vi "PCO_squeeze_puff_pupil_FLIR_trig_2024_JMR.vi"() -> ()   [LabVIEW 2020]
uses:
  C:/Users/jqr5792/AppData/Roaming/PCO Digital Camera Toolbox/pco.labview/pco.camera/Controls/binning.ctl
  <vilib>/vision/driver/IMAQdx.llb/IMAQdx Camera Control Mode.ctl
  <vilib>/userDefined/High Color/IMAQdx.ctl
  <vilib>/vision/driver/IMAQdx.llb/IMAQdx Acquisition Mode.ctl
  C:/Users/jqr5792/AppData/Roaming/PCO Digital Camera Toolbox/pco.labview/pco.camera/Camera.lvclass
  <vilib>/vision/driver/IMAQdx.llb/IMAQdx Buffer Number Mode.ctl
  7076c1c6-cf5a-4733-8e55-1dfd44238ec2.vi
  <vilib>/DAQmx/write.llb/DAQmx Write (Digital Bool 1Line 1Point).vi
  <vilib>/DAQmx/read.llb/DAQmx Read (Analog 1D Wfm NChan NSamp).vi
  <vilib>/DAQmx/write.llb/DAQmx Write (Digital 1D Bool NChan 1Samp 1Line).vi
  <vilib>/DAQmx/create/channels.llb/DAQmx Create Channel (AI-Voltage-Basic).vi
  <vilib>/DAQmx/configure/timing.llb/DAQmx Timing (Sample Clock).vi
  <vilib>/DAQmx/configure/trigger.llb/DAQmx Start Trigger (Digital Edge).vi
  <vilib>/DAQmx/create/channels.llb/DAQmx Create Channel (DO-Digital Output).vi
  <vilib>/DAQmx/create/channels.llb/DAQmx Create Channel (CO-Pulse Generation-Frequency).vi
  <vilib>/DAQmx/configure/timing.llb/DAQmx Timing (Implicit).vi
  <vilib>/DAQmx/miscellaneous.llb/DAQmx Fill In Error Info.vi
  <vilib>/vision/driver/NI_Vision_Acquisition_Software.lvlib
panel:
  out "New Lost":u32
  out "NewNumLost":u32[](array[numeric])
  out "NewBuffNum":u32[](array[numeric])
  out "Buffer Number Out":u32
  out "Min/Sec for trial":cluster{dbl, dbl}
  in  "Squeeze control duty cycle":dbl
  in  "Squeeze control freq (Hz)":dbl
  in  "Squeeze control":dbl=1.0
  in  "No stim":dbl=1.0
  in  "Peri-squeeze puff delay (s)":dbl=0.1 step=0.1
  in  "Squeeze \nDuration (s)":dbl=0.1 step=0.1
  out "n total images":i32
  out "PCO Frame Rate":dbl
  out "Time Elapsed (s)":u32
  out "Recorded Images":u32=7194
  out "PCO Recording":bool=TRUE
  in  "ROI":cluster{"x0":u64, "y0":u64, "x1":u64, "y1":u64}={"x0"=100, "y0"=175, "x1"=500, "y1"=425}
  in  "Binning":T1={"vert"=4, "horz"=4}
  in  "TriggerMode":T2(ring)=enum."external exposure start"
  in  "Exposure [s]":dbl=0.008 min=0.0005 max=2.0 step=0.001
  out "Image":T3(plugin-control)
  out "Last Whisk\nBuffer":u32=488
  out "Actual WhiskCam\nFrame Rate":dbl(knob)=148.05583250249254 scale=0.0..300.0
  out "Pupil":T3(plugin-control)
  out "Solenoids":bool[](array[boolean])
  in  "Stim \nOffset (s)":dbl=15.0
  in  "Puff \nDuration (s)":dbl=0.1 step=0.1
  in  "Inter-Stim\nInterval (s)":dbl=30.0
  in  "Stim and squeeze":dbl=1.0
  in  "Stim only":dbl=5.0
  in  "Squeeze only":dbl=2.0
  in  "Left Pad":tag="Dev1/port0/line1"
  in  "Right Pad":tag="Dev1/port0/line3"
  in  "Squeeze":tag="Dev1/port0/line2"
  out "Analog Data":bool
  out "Analog acquisition length":i32
  in  "Channel Labels":string[](array[string])=["BallVelocity", "LeftPad", "Control", "RightPad", "Broadband", "LFP", "MUA"]
  in  "physical channels":tag="Dev1/ai0:6"
  in  "Analog Acquisition Setup":cluster{"Analog Sampling Rate":u16}={"Analog Sampling Rate"=5000} {"Analog Sampling Rate" format="%0.0f"}
  in  "Camera Acquisition Setup":cluster{"CBVCam Rate":u16, "WebCam Rate":u16}={"CBVCam Rate"=60, "WebCam Rate"=30}
  out "Notes Size":i32=7
  out "Notes Reversed":string[](array[string])=["Experimenter", "Animal ID", "Imaged Hemisphere", "Solenoid Pressure", "Isoflurane time", "Session ID", "Amplifier Gain"]
  out "Notes Array":string[](array[string])=["Amplifier Gain", "Session ID", "Isoflurane time", "Solenoid Pressure", "Imaged Hemisphere", "Animal ID", "Experimenter"]
  in  "Session Notes:":T4={"Experimenter"="Joe Ricotta", "Animal ID"="T31", "Imaged Hemisphere"="RH", "Solenoid Pressure"="10", "Infusion Compound"="na", "Infusion volume nL"="na", "Infusion rate nlpS"="na", "Block"="1000", "Molar conc um"="na"}
  in  "Target Path":path=path "D:/Joe/sample/PCO_setup" caption="Final saved file location"
  out "Current file name":string="170828_12_37_58"
  out "Actual WebCam Frame Rate":dbl(knob) scale=0.0..30.0
  out "WebCam":T3(plugin-control)
  out "CBV Camera":bool=TRUE
  out "Trial Time Elapsed (Min)":cluster{dbl, dbl}(slide)={0.5, 0.05364406000000001} scale=0.0..20.0
  in  "Temp Path":path=path "C:/LabView Direct Files" caption="Temporary path for\nstreamed data"
  in  "Stop":bool
  # "File Settings:"
  # "2"
  # "Binning: 4,4"
  # "roi: 50, 200, 600, 400"
  # "10 of all stim"
  # "6"
  # "0.1"
  # "negative: puff precedes squeeze\nzero: puff and squeeze simultaneous\npositive: puff follows squeeze"
  # "Left Pad"
  # "Control"
  # "Right"
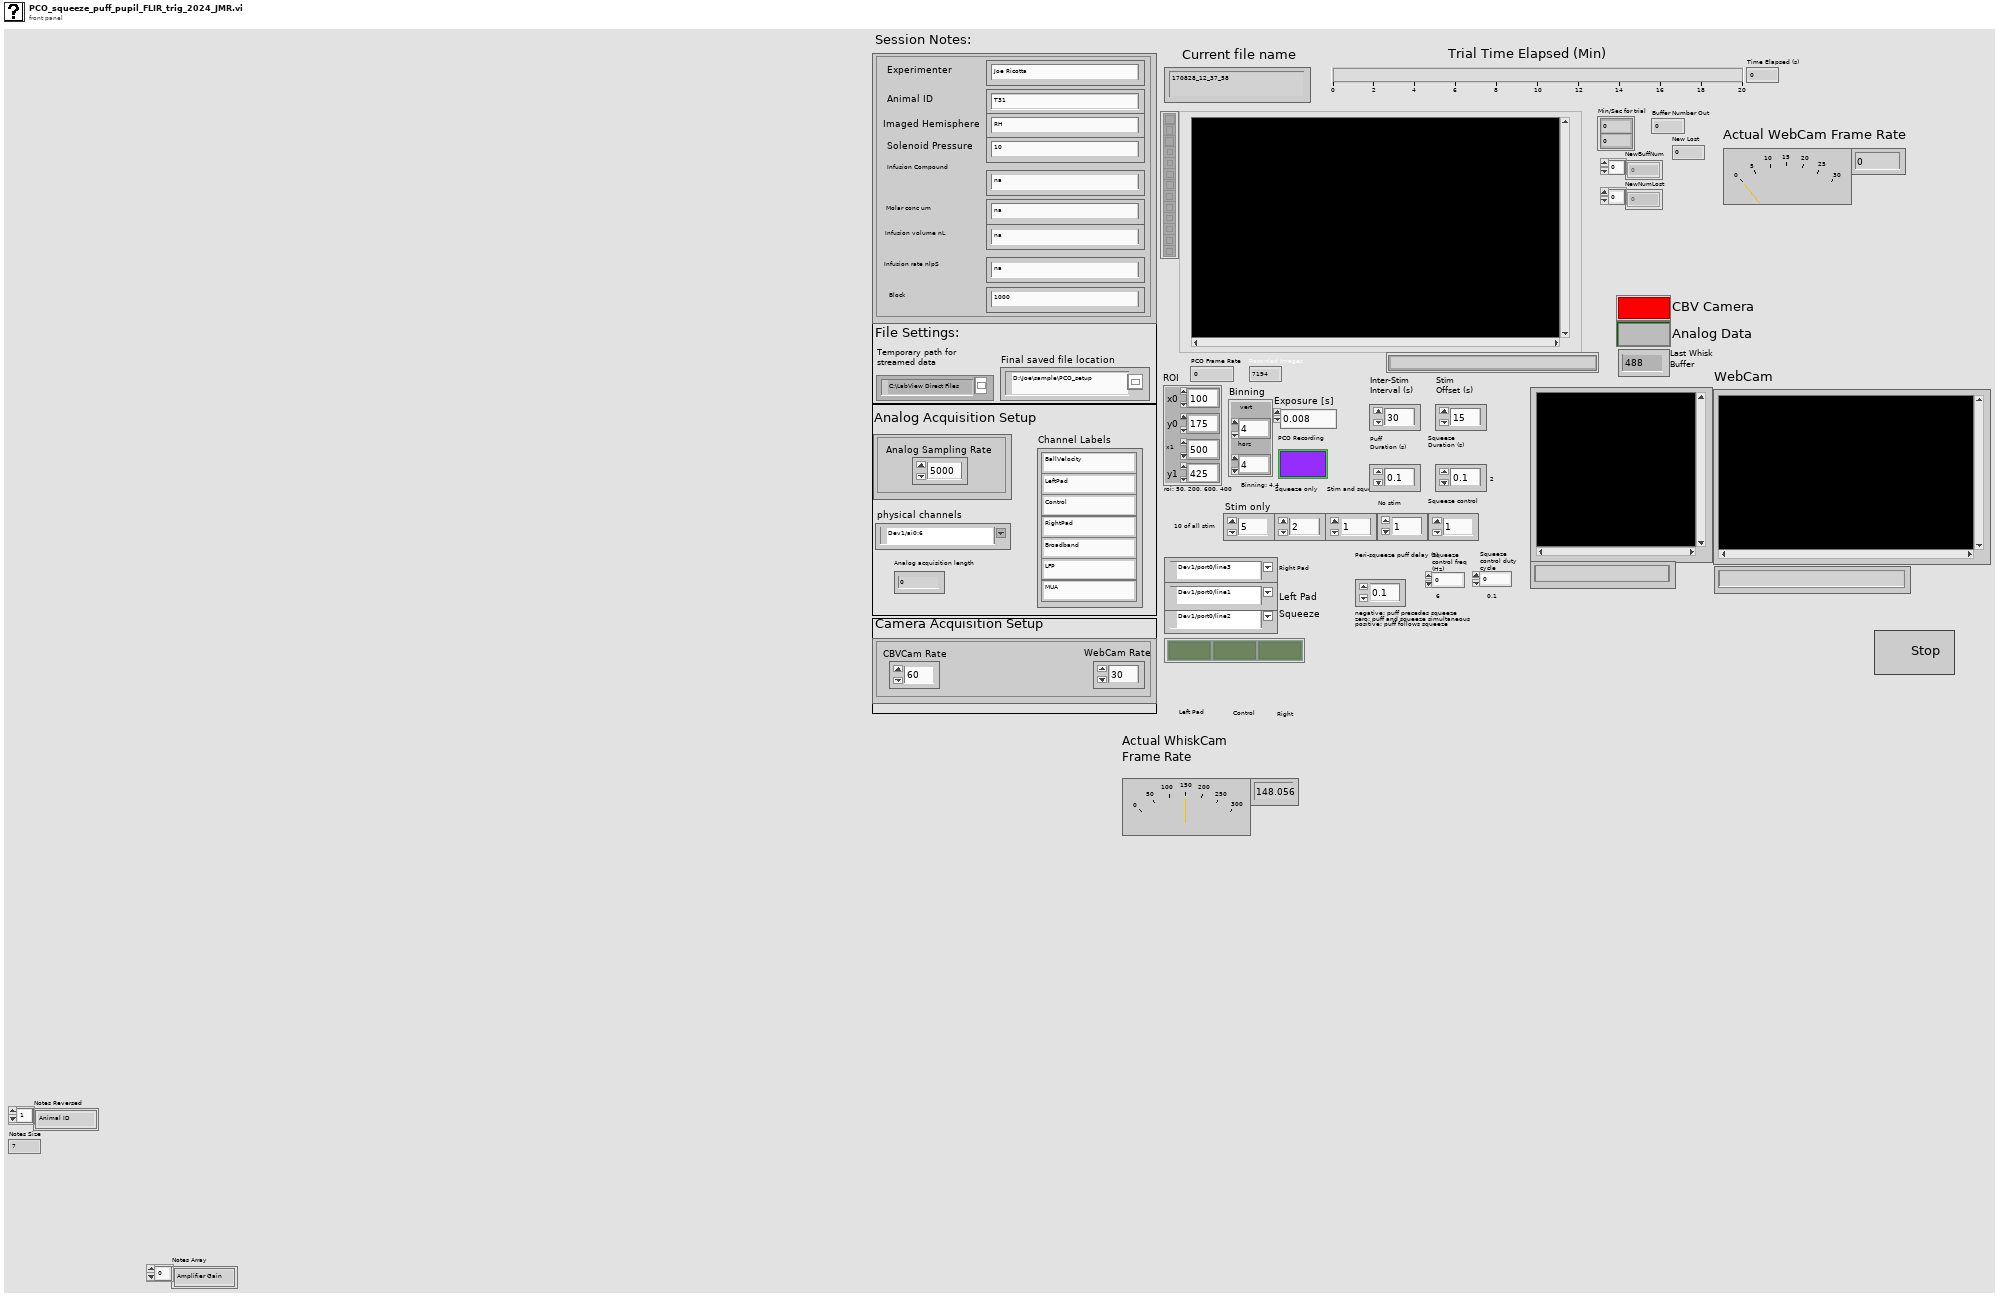
[diagram p1: front panel]
types:
  T1 = typedef "Camera.lvclass/binning.ctl" = cluster{"vert":u16, "horz":u16}
  T2 = enum16{"auto sequence", "software trigger", "external exposure start", "external exposure control"}
  T3 = typedef "IMAQ Image.ctl" = refnum<image>
  T4 = cluster{"Experimenter":string, "Animal ID":string, "Imaged Hemisphere":string, "Solenoid Pressure":string, "Infusion Compound":string, "Infusion volume nL":string, "Infusion rate nlpS":string, "Block":string, "Molar conc um":string}
  T5 = typedef "IMAQdx.ctl" = refnum<k21>
  T6 = typedef "Image Type" = u32
  T7 = enum16{"open", "replace", "create", "open or create", "replace or create", "replace or create with confirmation"}
  T8 = typedef "NI_Vision_Acquisition_Software.lvlib/IMAQdx Acquisition Mode.ctl" = enum32{"One Shot", "Continuous"}
  T9 = typedef "NI_Vision_Acquisition_Software.lvlib/IMAQdx Camera Control Mode.ctl" = enum32{"Controller", "Listener"}
  T10 = enum16{"open", "open or create", "create or replace", "create", "open (read-only)"}
  T11 = cluster{"exposure_time_s":dbl, "delay_time_s":dbl, "roi":cluster{"x0":u64, "y0":u64, "x1":u64, "y1":u64}, "timestamp_mode":u16, "pixelrate":u32, "trigger_mode":u16, "acquire_mode":u16, "metadata_mode":u16, "noisefilter_mode":u16, "binning":T1}
  T12 = typedef "IMAQ AVI2 Refnum.ctl" = refnum<k20>
  T13 = enum16{"sequence", "sequence non blocking", "ring buffer", "fifo", "sequence_dpcore", "sequence_non_blocking_dpcore", "ring_buffer_dpcore", "fifo_dpcore", "tif", "multitif", "pcoraw", "b16", "dicom", "multidicom"}
  T14 = enum16{"Undefined", "Mono8", "Mono16", "BGRA8", "RGBA8", "BGRA16", "RGBA16", "CompressedMono8"}
  T15 = enum16{"big-endian, network order", "native, host order", "little-endian"}
  T16 = typedef "NI_Vision_Acquisition_Software.lvlib/IMAQdx Buffer Number Mode.ctl" = enum32{"Next", "Last", "Buffer Number", "Every", "Last New"}
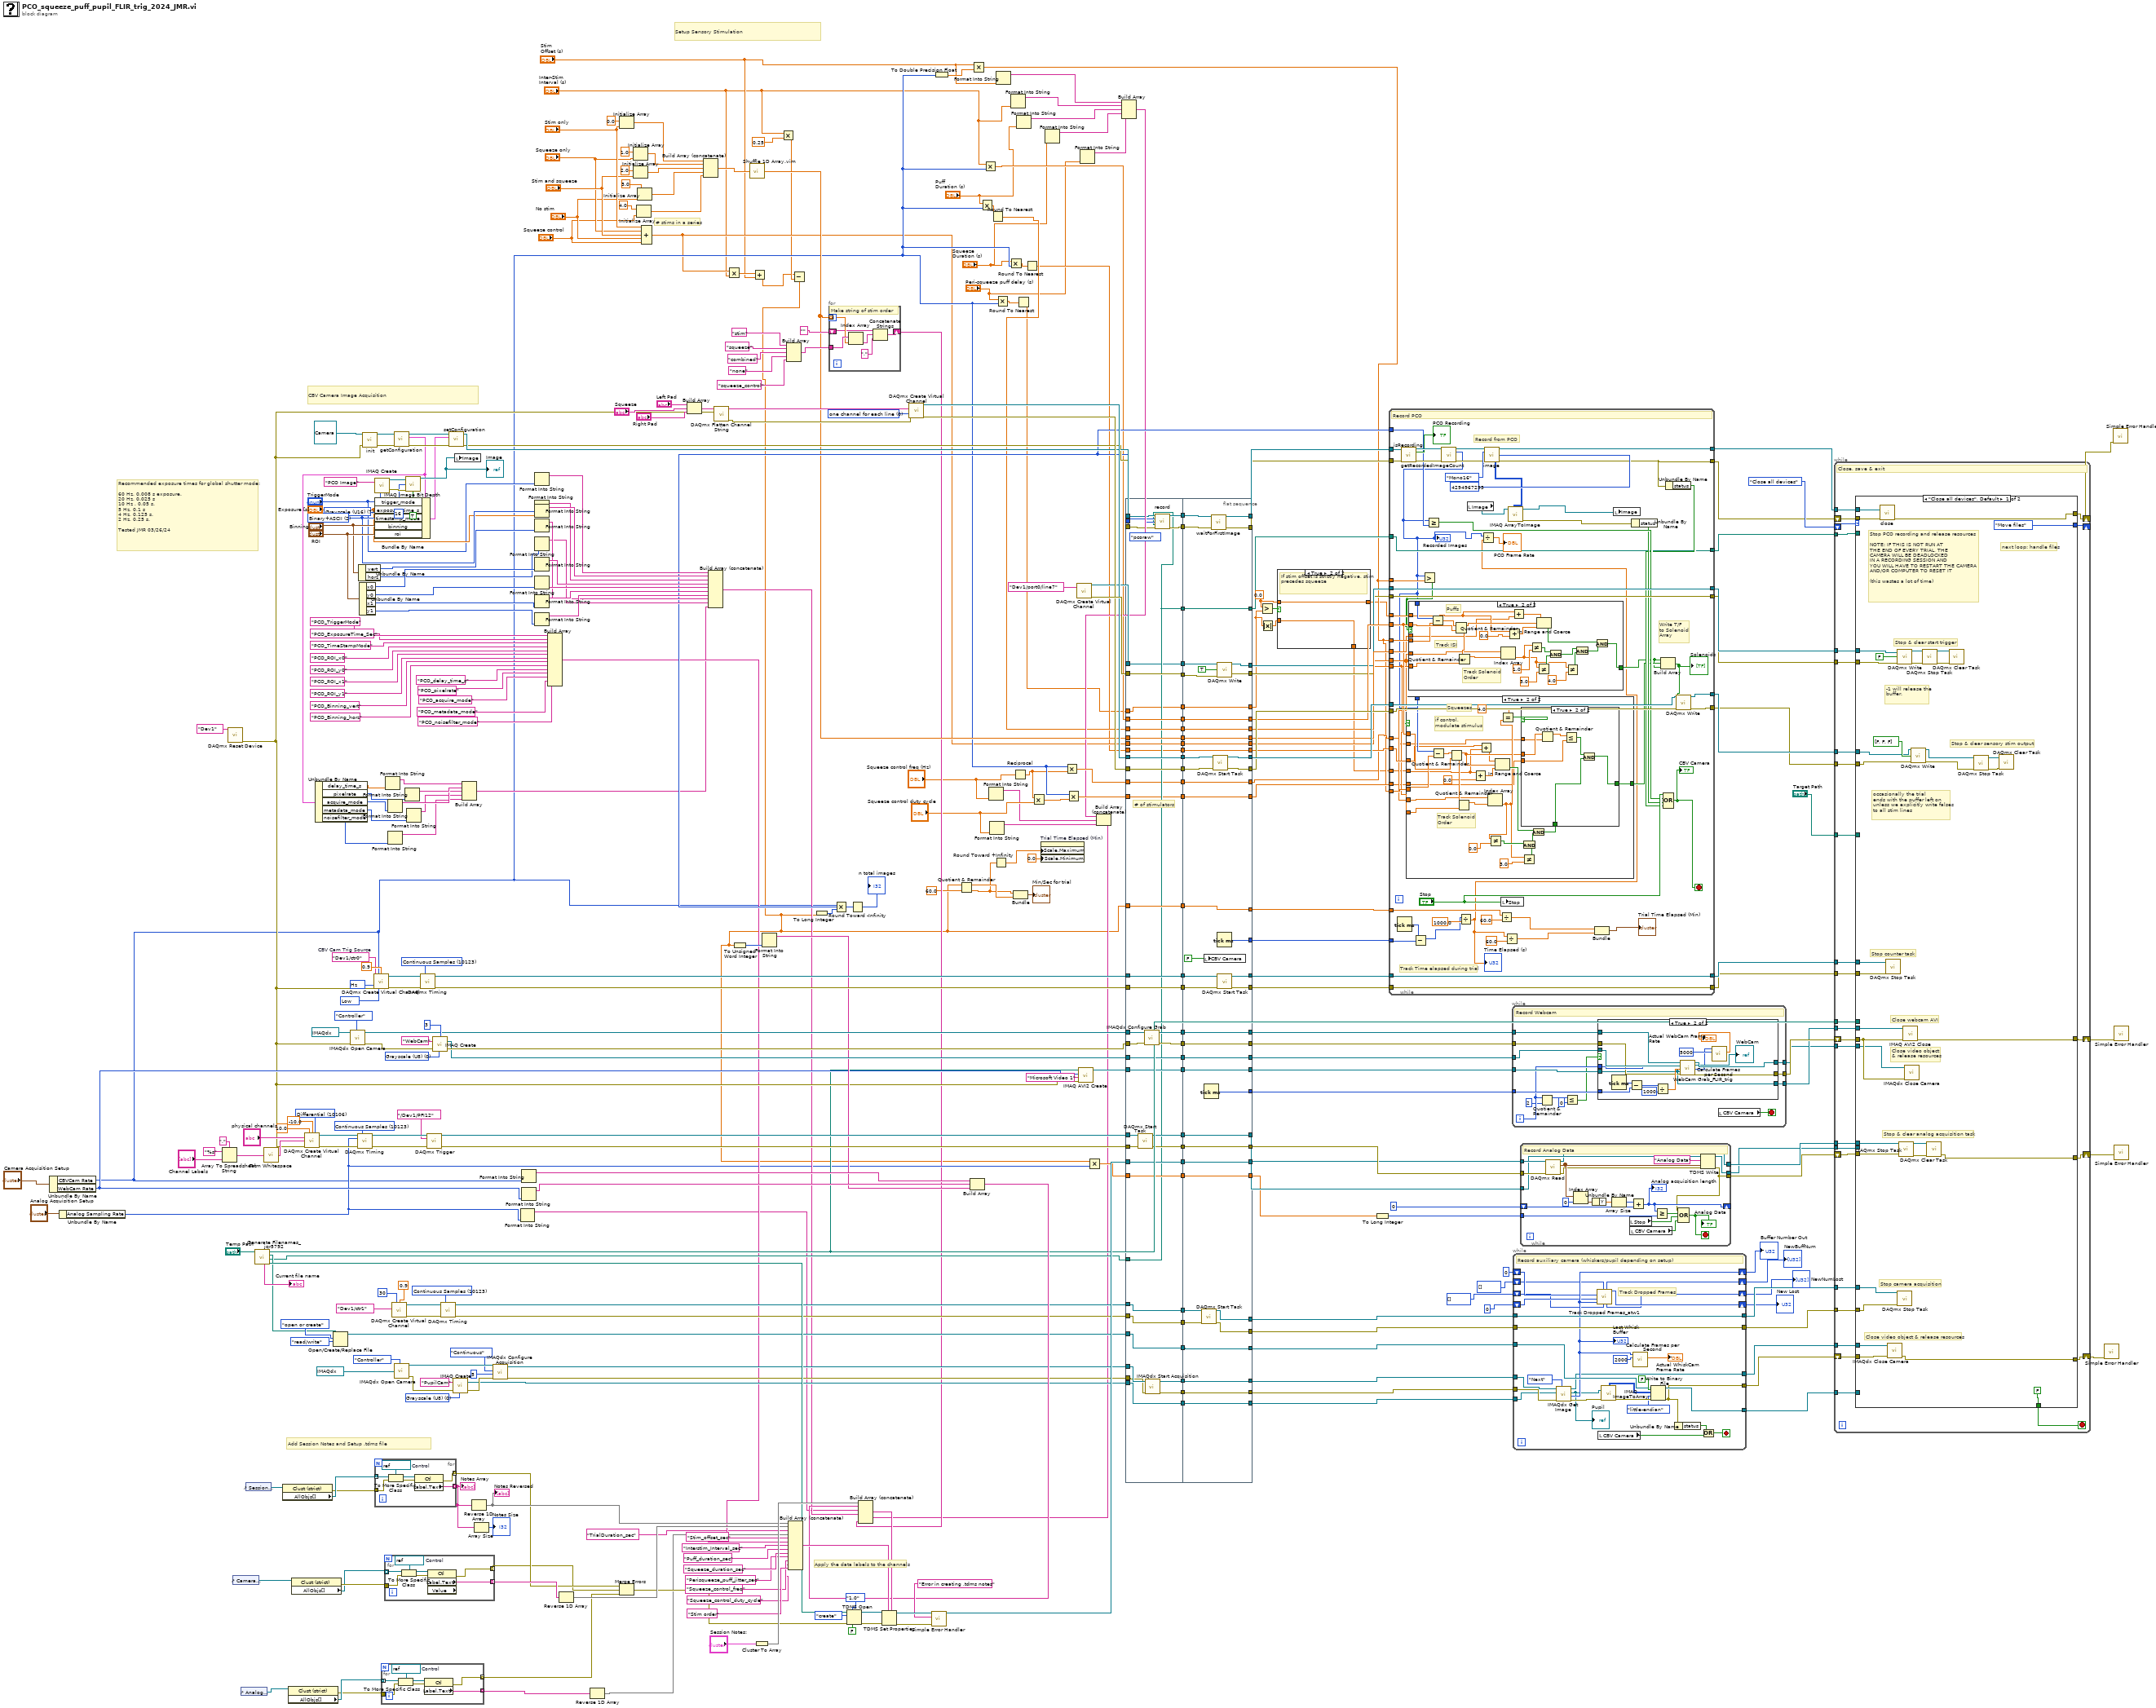
[diagram p0: block diagram]
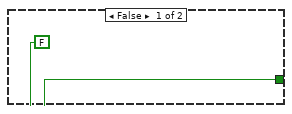
[diagram p3: hidden frame]
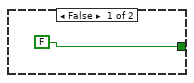
[diagram p5: hidden frame]
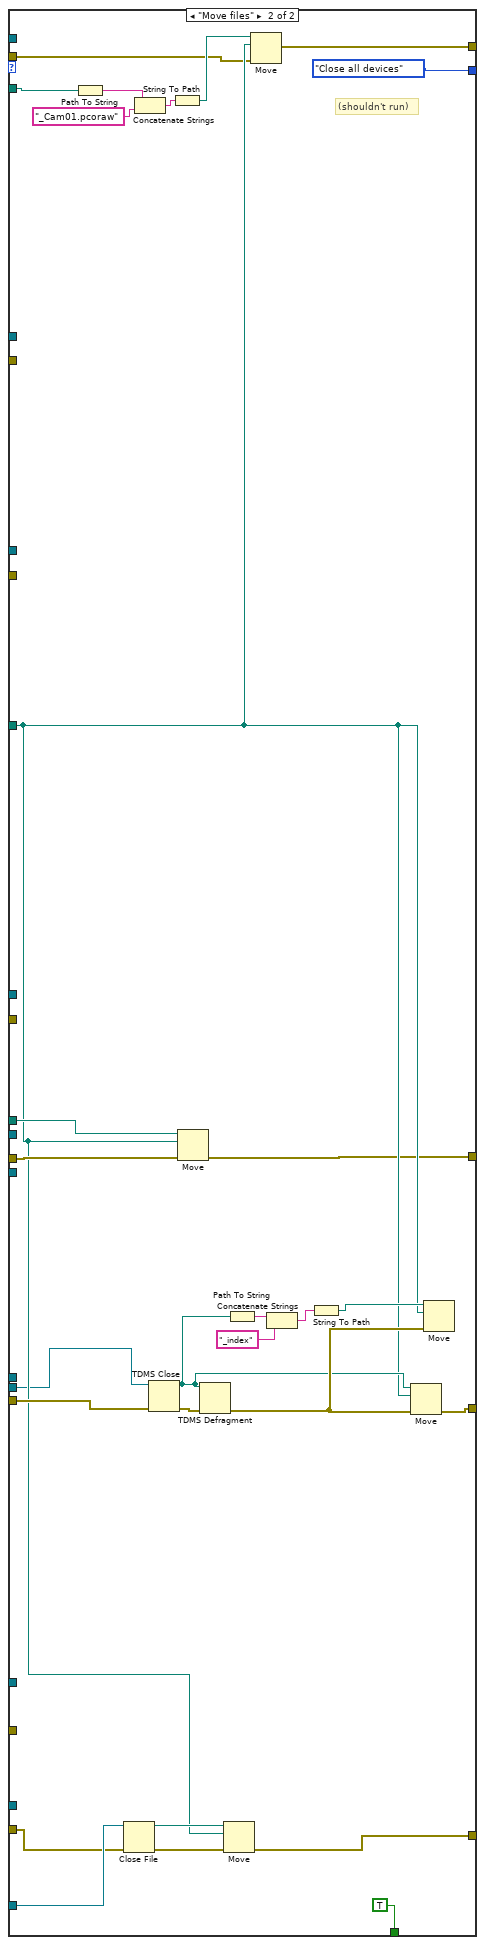
[diagram p6: hidden frame]
diagram:
  w5 = 0.0 ("y")
  w157 = u16 2 items=["OFF", "Binary", "Binary+ASCII", "ASCII"] ("wTimeStampMode")
  w188 = T6 7 items=["Grayscale (U8)", "Grayscale (I16)", "Grayscale (SGL)", "Complex (CSG)", "RGB (U32)", "HSL (U32)", "RGB (U64)", "Grayscale (U16)"] ("Image Type")
  w218 = 10123 items=["Finite Samples"=10178, "Continuous Samples"=10123, "Hardware Timed Single Point"=12522] ("sample mode")
  w223 = T6 0 items=["Grayscale (U8)", "Grayscale (I16)", "Grayscale (SGL)", "Complex (CSG)", "RGB (U32)", "HSL (U32)", "RGB (U64)", "Grayscale (U16)"] ("Image Type")
  w264 = 0 items=["one channel for each line", "one channel for all lines"] ("line grouping")
  w267 = tag "Dev1/ctr0"  # CBV Cam Trig Source
  w340 = 10123 items=["Finite Samples"=10178, "Continuous Samples"=10123, "Hardware Timed Single Point"=12522] ("sample mode")
  w343 = 10106 items=["default"=-1, "RSE"=10083, "NRSE"=10078, "Differential"=10106, "Pseudodifferential"=12529] ("input terminal configuration")
  w363 = T6 0 items=["Grayscale (U8)", "Grayscale (I16)", "Grayscale (SGL)", "Complex (CSG)", "RGB (U32)", "HSL (U32)", "RGB (U64)", "Grayscale (U16)"] ("Image Type")
  w368 = 10123 items=["Finite Samples"=10178, "Continuous Samples"=10123, "Hardware Timed Single Point"=12522] ("sample mode")
  w371 = 10373 items=["Hz"=10373] ("units")
  w372 = 10214 items=["High"=10192, "Low"=10214] ("idle state")
  # "Recommended exposure times for global shutter mode:\n\n60 Hz, 0.008 s exposure.\n20 Hz, 0.025 s\n10 Hz , 0.05 s.\n5 Hz, 0.1 s\n4 Hz, 0.125 s.\n2 Hz, 0.25 s.\n\nTested JMR 03/26/24"
  # "Setup Sensory Stimulation"
  # "# stims in a series"
  # "Apply the data labels to the channels"
  # "CBV Camera Image Acquisition"
  # "Add Session Notes and Setup .tdms file"
  n1 = Unbundle By Name "Unbundle By Name"("Camera Acquisition Setup") -> ("CBVCam Rate"=w48:u16, "WebCam Rate"=w194:u16)
  n2 = Unbundle By Name("Analog Acquisition Setup") -> ("Analog Sampling Rate"=w104:u16)
  n3 = Array To Spreadsheet String(delimiter (Tab)=",", array="Channel Labels", 3:"%s" ("format string")) -> (spreadsheet string=w281:string)
  n4 = call <vilib>:"DAQmx Reset Device.vi"("device in"=tag "Dev1") -> ("error out"=w140:errorcluster)  [unwired: 14 in]
  n5 = control-ref of="Camera Acquisition Setup"() -> (w294:refnum<vi>)
  n6 = control-ref of="Analog Acquisition Setup"() -> (w293:refnum<vi>)
  n7 = control-ref of="Session Notes:"() -> (w317:refnum<vi>)
  n8 = call "Generate Filenames_jqr5792.vi"("path"="Temp Path") -> ("TDMS Path"=w311:path, "PCO Path"=w150:path, "Basler Path"=w215:path, "WebCam Path"=w118:path, "Analog file name"=→"Current file name":string)  [unwired: 5 in, 1 out]
  n9 = call <vilib>:"Trim Whitespace.vi"("string"=w281) -> ("trimmed string"=w280:string)  [unwired: 1 in]
  n10 = property class="Clust (strict)"(reference=w317) -> (error out=w320:errorcluster, "AllObjs[]"=w321:refnum<vi>[])  [unwired: 1 in, 1 out]
  n11 = property class="Clust (strict)"(reference=w293) -> (error out=w291:errorcluster, "AllObjs[]"=w292:refnum<vi>[])  [unwired: 1 in, 1 out]
  n12 = property class="Clust (strict)"(reference=w294) -> (error out=w315:errorcluster, "AllObjs[]"=w314:refnum<vi>[])  [unwired: 1 in, 1 out]
  n13 = call-poly <vilib>:"DAQmx Create Virtual Channel.vi"("maximum value"=10.0, "minimum value"=-10.0, "input terminal configuration"=w343, "physical channels"="physical channels", "name to assign"=w280, "error in"=w140) -> ("task out"=w342:refnum<k21>, "error out"=w341:errorcluster)  [unwired: 8 in]
  n14 = Open/Create/Replace File(file path (use dialog)=w215, operation (0:open)=T7."open or create", access (0:read/write)=enum16{"read/write", "read-only", "write-only"}."read/write") -> (refnum out=w199:refnum<file>)  [unwired: 3 in, 2 out]
  n15 = call <vilib>:"IMAQdx Open Camera.vi"("Camera Control Mode"=IMAQdx_Camera_Control_Mode."Controller", "error in"=w140, "Session In"=T5 "cam9") -> ("error out"=w360:errorcluster, "Session Out"=w358:T5)  [unwired: 7 in]
  n16 = call-poly <vilib>:"DAQmx Timing.vi"("task/channels in"=w342, "sample mode"=w340, "rate"=w104, "error in"=w341) -> ("task out"=w339:refnum<k21>, "error out"=w338:errorcluster)  [unwired: 10 in]
  n17 = Unbundle By Name("Binning") -> ("vert"=w158:u16, "horz"=w159:u16)
  n18 = Unbundle By Name("ROI") -> ("x0"=w160:u64, "y0"=w161:u64, "x1"=w162:u64, "y1"=w163:u64)
  n19 = call-dynamic "init.vi"("Camera in"=refnum<class "Camera.lvclass"> refnum ("PCOCamera in"), "error in (no error)"=w140) -> ("Camera out"=w185:refnum<class "Camera.lvclass">, "error out"=w184:errorcluster)  [unwired: 7 in]
  n20 = call-poly <vilib>:"DAQmx Create Virtual Channel.vi"("frequency"=w48, "duty cycle"=0.9, "counter"=w267, "units"=w371, "error in"=w140, "idle state"=w372) -> ("task out"=w370:refnum<k21>, "error out"=w369:errorcluster)  [unwired: 8 in]
  n21 = call "IMAQ Create"("Image Name"="PCO Image", "Image Type"=w188) -> ("New Image"=w73:T3, "error out"=w187:errorcluster)  [unwired: 3 in]
  n22 = for {
    tunnel: [w377] -> w319 mode=indexing
    tunnel: w321 -> [w376] mode=indexing
    tunnel: w320 -> [w375]
    tunnel: [w373] -> w300 mode=indexing
    w378 = refnum<vi> refnum  # Control
    n23 = To More Specific Class(target class=w378, reference=w376, error in=w375) -> (specific class reference=w379:refnum<vi>, error out=w374:errorcluster)
    n24 = property class="Ctl"(reference=w379, error in=w374) -> (error out=w373:errorcluster, "Label.Text"=w377:string)  [unwired: 1 out]
  }
  "Notes Array" <- w319
  n25 = for {
    tunnel: [w384] -> w289 mode=indexing
    tunnel: w292 -> [w383] mode=indexing
    tunnel: w291 -> [w382]
    tunnel: [w380] -> w290 mode=indexing
    w385 = refnum<vi> refnum  # Control
    n26 = To More Specific Class(target class=w385, reference=w383, error in=w382) -> (specific class reference=w386:refnum<vi>, error out=w381:errorcluster)
    n27 = property class="Ctl"(reference=w386, error in=w381) -> (error out=w380:errorcluster, "Label.Text"=w384:string)  [unwired: 1 out]
  }
  n28 = for {
    tunnel: [w391] -> w316 mode=indexing
    tunnel: w314 -> [w390] mode=indexing
    tunnel: w315 -> [w389]
    tunnel: [w387] -> w299 mode=indexing
    w392 = refnum<vi> refnum  # Control
    n29 = To More Specific Class(target class=w392, reference=w390, error in=w389) -> (specific class reference=w393:refnum<vi>, error out=w388:errorcluster)
    n30 = property class="Ctl" props=["Label", "Text", "Value"](reference=w393, error in=w388) -> (error out=w387:errorcluster, "Label.Text"=w391:string)  [unwired: 2 out]
  }
  n31 = call-poly <vilib>:"DAQmx Create Virtual Channel.vi"("frequency"=30, "duty cycle"=0.9, "counter"=tag "Dev1/ctr1" ("Whisker Cam\nTrigger Source")) -> ("task out"=w220:refnum<k21>, "error out"=w219:errorcluster)  [unwired: 11 in]
  n32 = call-dynamic "getConfiguration.vi"("error in (no error)"=w184, "Camera in"=w185) -> ("error out"=w183:errorcluster, "configuration"=w102:T11, "Camera out"=w186:refnum<class "Camera.lvclass">)  [unwired: 7 in]
  n33 = Unbundle By Name(w102) -> ("delay_time_s"=w96:dbl, "pixelrate"=w95:u32, "acquire_mode"=w94:u16, "metadata_mode"=w93:u16, "noisefilter_mode"=w92:u16)
  n34 = Bundle By Name(cluster=w102, "trigger_mode"="TriggerMode", "exposure_time_s"="Exposure [s]", "timestamp_mode"=w157, "binning"="Binning", "roi"="ROI") -> (w182:T11)
  n35 = Format Into String(w96) -> (resulting string=w91:string)  [unwired: 3 in, 1 out]
  n36 = Format Into String(w92) -> (resulting string=w87:string)  [unwired: 3 in, 1 out]
  n37 = Format Into String(w94) -> (resulting string=w89:string)  [unwired: 3 in, 1 out]
  n38 = call <vilib>:"IMAQdx Open Camera.vi"("Camera Control Mode"=IMAQdx_Camera_Control_Mode."Controller", "Session In"=T5 "cam5" ("Pupil Cam")) -> ("error out"=w226:errorcluster, "Session Out"=w229:T5)  [unwired: 8 in]
  n39 = Format Into String(w95) -> (resulting string=w90:string)  [unwired: 3 in, 1 out]
  n40 = call "IMAQ Image Bit Depth"("Image"=w73, "Bit Depth (0)"=u32 16, "error in (no error)"=w187, "Get/Set Bit Depth? (Set)"=TRUE) -> ("Image Out"=w189:T3)  [unwired: 9 in, 2 out]
  "Image" <- w189
  n41 = Format Into String(w93) -> (resulting string=w88:string)  [unwired: 3 in, 1 out]
  n42 = call-poly <vilib>:"DAQmx Timing.vi"("task/channels in"=w370, "sample mode"=w368, "error in"=w369) -> ("task out"=w327:refnum<k21>, "error out"=w325:errorcluster)  [unwired: 11 in]
  n43 = call-poly <vilib>:"DAQmx Trigger.vi"("task/channels in"=w339, "source"=tag "/Dev1/PFI12", "error in"=w338) -> ("task out"=w336:refnum<k21>, "error out"=w335:errorcluster)  [unwired: 11 in]
  n44 = call "IMAQ Create"("Border Size"=3, "Image Name"="WebCam", "Image Type"=w363, "error in (no error)"=w360) -> ("New Image"=w357:T3, "error out"=w359:errorcluster)  [unwired: 1 in]
  n45 = call-poly <vilib>:"DAQmx Timing.vi"("task/channels in"=w220, "sample mode"=w218, "error in"=w219) -> ("task out"=w208:refnum<k21>, "error out"=w206:errorcluster)  [unwired: 11 in]
  n46 = call-dynamic "setConfiguration.vi"("error in (no error)"=w183, "configuration"=w182, "Camera in"=w186) -> ("error out"=w151:errorcluster, "Camera out"=w152:refnum<class "Camera.lvclass">)  [unwired: 7 in]
  n47 = call "IMAQ Create"("Image Name"="PupilCam", "Image Type"=w223, "error in (no error)"=w226) -> ("New Image"=w202:T3, "error out"=w224:errorcluster)  [unwired: 2 in]
  n48 = local write "Image"(w189) -> ()
  n49 = Build Array(w91, w90, w89, w88, w87) -> (w86:string[])
  n50 = Reverse 1D Array(array=w319) -> (reversed array=w305:string[])
  "Notes Reversed" <- w305
  n51 = Array Size(array=w319) -> (size(s)=→"Notes Size":i32)
  n52 = call <vilib>:"IMAQdx Configure Acquisition.vi"("error in"=w224, "Number of Buffers"=u32 5, "Continuous?"=IMAQdx_Acquisition_Mode."Continuous", "Session In"=w229) -> ("error out"=w203:errorcluster, "Session Out"=w204:T5)  [unwired: 6 in]
  n53 = Format Into String(w104) -> (resulting string=w103:string)  [unwired: 3 in, 1 out]
  n54 = Format Into String(w48) -> (resulting string=w287:string)  [unwired: 3 in, 1 out]
  n55 = Format Into String(w194) -> (resulting string=w286:string)  [unwired: 3 in, 1 out]
  n56 = Format Into String("TriggerMode") -> (resulting string=w170:string)  [unwired: 3 in, 1 out]
  n57 = Format Into String(w157) -> (resulting string=w168:string)  [unwired: 3 in, 1 out]
  n58 = Format Into String("Exposure [s]") -> (resulting string=w169:string)  [unwired: 3 in, 1 out]
  n59 = Format Into String(w158) -> (resulting string=w154:string)  [unwired: 3 in, 1 out]
  n60 = Format Into String(w159) -> (resulting string=w153:string)  [unwired: 3 in, 1 out]
  n61 = Format Into String(w160) -> (resulting string=w167:string)  [unwired: 3 in, 1 out]
  n62 = Format Into String(w161) -> (resulting string=w166:string)  [unwired: 3 in, 1 out]
  n63 = Format Into String(w162) -> (resulting string=w165:string)  [unwired: 3 in, 1 out]
  n64 = Format Into String(w163) -> (resulting string=w164:string)  [unwired: 3 in, 1 out]
  n65 = Build Array("PCO_TriggerMode", "PCO_ExposureTime_Sec", "PCO_TimeStampMode", "PCO_ROI_x0", "PCO_ROI_y0", "PCO_ROI_x1", "PCO_ROI_y1", "PCO_Binning_vert", "PCO_Binning_horz", "PCO_delay_time_s", "PCO_pixelrate", "PCO_acquire_mode", "PCO_metadata_mode", "PCO_noisefilter_mode") -> (w108:string[])
  n66 = Reverse 1D Array(array=w316) -> (reversed array=w304:string[])
  n67 = Reverse 1D Array(array=w289) -> (reversed array=w288:string[])
  n68 = Initialize Array(0.0 ("element"), "Stim only") -> (w260:dbl[])
  n69 = Merge Errors(w300, w299, w290) -> (w298:errorcluster)
  n70 = Initialize Array(1.0 ("element"), "Squeeze only") -> (w259:dbl[])
  n71 = Initialize Array(2.0 ("element"), "Stim and squeeze") -> (w258:dbl[])
  n72 = Initialize Array(4.0 ("element"), "Squeeze control") -> (w53:dbl[])
  n73 = Initialize Array(3.0 ("element"), "No stim") -> (w64:dbl[])
  n74 = Compound Arithmetic op=ADD("Stim only", "Squeeze only", "Stim and squeeze", "No stim", "Squeeze control") -> (w33:dbl)
  n75 = Build Array("Left Pad", "Squeeze", "Right Pad") -> (w265:tag[])
  n76 = Build Array (concatenate)(w260, w259, w258, w64, w53) -> (w74:dbl[])
  n77 = Build Array (concatenate)(w170, w169, w168, w167, w166, w165, w164, w154, w153, w86) -> (w107:string[])
  n78 = call <vilib>:"DAQmx Flatten Channel String.vi"("names in"=w265, "error in"=w140) -> ("names out"=w238:string, "error out"=w239:errorcluster)  [unwired: 12 in]
  n79 = Multiply(x=w33, y="Inter-Stim\nInterval (s)") -> (x*y=w32:dbl)
  n80 = call "Shuffle 1D Array.vim"("array"=w74) -> ("shuffled array"=w57:dbl[])  [unwired: 4 in]
  n81 = Add(x=w32, y="Stim \nOffset (s)") -> (x+y=w23:dbl)
  n82 = Cluster To Array(cluster="Session Notes:") -> (array=w312:string[])
  n83 = Multiply(x="Inter-Stim\nInterval (s)", y=0.25) -> (x*y=w24:dbl)
  n84 = Build Array("stim", "squeeze", "combined", "none", "squeeze_control") -> (w59:string[])
  n85 = Build Array (concatenate)(w305, w304, "TrialDuration_sec", w288, w108, "Stim_offset_sec" ("array"), "Interstim_Interval_sec" ("array"), "Puff_duration_sec" ("array"), "Squeeze_duration_sec" ("array"), "Perisqueeze_puff_jitter_sec" ("array"), "Squeeze_control_freq" ("array"), "Squeeze_control_duty_cycle" ("array"), "Stim order" ("array")) -> (w302:string[])
  n86 = Subtract(x=w23, y=w24) -> (x-y=w22:dbl)
  n87 = To Unsigned Word Integer(number=w22) -> (unsigned 16bit integer=w277:u16)
  n88 = Format Into String(w277) -> (resulting string=w278:string)  [unwired: 3 in, 1 out]
  n89 = To Long Integer(number=w22) -> (32bit integer=w145:i32)
  n90 = for {
    tunnel: w59 -> [w399]
    shift-right: [w396] -> w56
    shift-left: "" -> [w395]
    tunnel: w57 -> [w398] mode=indexing
    # "Make string of stim order"
    n91 = Index Array(array=w399, index=w398) -> (element=w397:string)
    n92 = Concatenate Strings(w395, w397, "," ("string")) -> (w396:string)
  }
  n93 = Multiply(x=w48, y=w145) -> (x*y=w144:i32)
  n94 = TDMS Open(6:FALSE ("disable buffering? (T)"), 7:enum16{"1.0", "2.0"}."1.0" ("file format version (2.0)"), 8:w298, 10:T10."create" ("operation (0:open)"), 11:w311) -> (0:w306:errorcluster, 3:w307:refnum<k34>)  [unwired: 2 in]
  n95 = Round Toward -Infinity(1:w144) -> (0:w143:i32)
  "n total images" <- w143
  n96 = call-poly <vilib>:"DAQmx Create Virtual Channel.vi"("lines"=w238, "line grouping"=w264, "error in"=w239) -> ("task out"=w254:refnum<k21>, "error out"=w252:errorcluster)  [unwired: 11 in]
  n97 = To Double Precision Float(number=w48) -> (double precision float=w256:dbl)
  n98 = Quotient & Remainder(x=w22, y=60.0) -> (x-y*floor(x/y)=w31:dbl, floor(x/y)=w28:dbl)
  n99 = Build Array(w287, w286, w278) -> (w285:string[])
  n100 = Multiply(x="Stim \nOffset (s)", y=w256) -> (x*y=w20:dbl)
  n101 = Multiply(x="Puff \nDuration (s)", y=w48) -> (x*y=w257:dbl)
  n102 = Multiply(x="Inter-Stim\nInterval (s)", y=w48) -> (x*y=w18:dbl)
  n103 = Format Into String("Squeeze control freq (Hz)") -> (resulting string=w39:string)  [unwired: 3 in, 1 out]
  n104 = Format Into String("Squeeze control duty cycle") -> (resulting string=w38:string)  [unwired: 3 in, 1 out]
  n105 = Round To Nearest(number=w257) -> (nearest integer value=w16:dbl)
  n106 = Round Toward +Infinity(x=w28) -> (ceil(x): smallest int >= x=w27:dbl)
  n107 = Multiply(x="Peri-squeeze puff delay (s)", y=w48) -> (x*y=w78:dbl)
  n108 = Format Into String("Stim \nOffset (s)") -> (resulting string=w82:string)  [unwired: 3 in, 1 out]
  n109 = Multiply(x="Squeeze \nDuration (s)", y=w48) -> (x*y=w79:dbl)
  n110 = Format Into String("Inter-Stim\nInterval (s)") -> (resulting string=w81:string)  [unwired: 3 in, 1 out]
  n111 = Reciprocal(x="Squeeze control freq (Hz)") -> (1/x=w43:dbl)
  n112 = Bundle(w28, w31) -> (→"Min/Sec for trial":cluster{dbl, dbl})  [unwired: 1 in]
  n113 = Format Into String("Puff \nDuration (s)") -> (resulting string=w80:string)  [unwired: 3 in, 1 out]
  n114 = Round To Nearest(number=w78) -> (nearest integer value=w12:dbl)
  n115 = Round To Nearest(number=w79) -> (nearest integer value=w14:dbl)
  n116 = Multiply(x=w43, y="Squeeze control duty cycle") -> (x*y=w47:dbl)
  n117 = property on="Trial Time Elapsed (Min)" class="Slide (strict)"("Scale.Maximum"=w27, "Scale.Minimum"=0.0 ("Scale.Range:Minimum")) -> ()  [unwired: 2 in, 2 out]
  n118 = Format Into String("Squeeze \nDuration (s)") -> (resulting string=w68:string)  [unwired: 3 in, 1 out]
  n119 = Multiply(x=w48, y=w43) -> (x*y=w49:dbl)
  n120 = Multiply(x=w48, y=w47) -> (x*y=w46:dbl)
  n121 = call-poly <vilib>:"DAQmx Create Virtual Channel.vi"("lines"=tag "Dev1/port0/line7") -> ("task out"=w137:refnum<k21>, "error out"=w270:errorcluster)  [unwired: 13 in]
  n122 = call "IMAQ AVI2 Create"("error in (no error)"=w140, "Codec"="Microsoft Video 1", "Frames Per Second"=w194, "AVI Path"=w118) -> ("AVI Refnum"=w193:T12)  [unwired: 6 in, 1 out]
  n123 = Format Into String("Peri-squeeze puff delay (s)") -> (resulting string=w67:string)  [unwired: 3 in, 1 out]
  n124 = Multiply(x=w22, y=w104) -> (x*y=w275:dbl)
  n125 = Build Array(w82, w81, w80, w68, w67) -> (w40:string[])
  n126 = Build Array (concatenate)(w40, w39, w38) -> (w37:string[])
  n127 = Build Array (concatenate)(w312, w285, w103, w107, w37, w56) -> (w303:string[])
  n128 = TDMS Set Properties(5:w303, 7:w302, 8:w306, 11:w307) -> (0:w297:errorcluster, 3:w301:refnum<k34>)  [unwired: 2 in, 2 out]
  n129 = call <vilib>:"Simple Error Handler.vi"("error source (\" \")"="Error in creating .tdms notes" ("error source (\" \")"), "error in (no error)"=w297) -> ()  [unwired: 3 in, 5 out]
  n130 = flat-sequence {
    tunnel: w359 -> [w441]
    tunnel: w358 -> [w440]
    tunnel: w357 -> [w439]
    tunnel: [w439] -> w356
    tunnel: [w438] -> w354
    tunnel: [w437] -> w352
    tunnel: w193 -> [w436]
    tunnel: [w436] -> w350
    tunnel: w22 -> [w435]
    tunnel: [w435] -> w344
    tunnel: w336 -> [w434]
    tunnel: w335 -> [w433]
    tunnel: [w432] -> w334
    tunnel: [w431] -> w333
    tunnel: [w430] -> w328
    tunnel: w301 -> [w430]
    tunnel: w327 -> [w429]
    tunnel: [w429] -> w326
    tunnel: w325 -> [w428]
    tunnel: [w428] -> w324
    tunnel: w275 -> [w427]
    tunnel: [w427] -> w274
    tunnel: w270 -> [w426]
    tunnel: [w426] -> w269
    tunnel: w254 -> [w425]
    tunnel: [w425] -> w253
    tunnel: w252 -> [w424]
    tunnel: [w424] -> w251
    tunnel: [w423] -> w247
    tunnel: w18 -> [w423]
    tunnel: w16 -> [w422]
    tunnel: [w422] -> w246
    tunnel: w57 -> [w421]
    tunnel: [w421] -> w244
    tunnel: w33 -> [w420]
    tunnel: [w420] -> w242
    tunnel: [w419] -> w212
    tunnel: [w418] -> w210
    tunnel: w208 -> [w417]
    tunnel: [w417] -> w207
    tunnel: w206 -> [w416]
    tunnel: [w416] -> w205
    tunnel: w204 -> [w415]
    tunnel: [w414] -> _
    tunnel: w203 -> [w414]
    tunnel: w202 -> [w413]
    tunnel: [w413] -> w201
    tunnel: w199 -> [w412]
    tunnel: [w412] -> w198
    tunnel: w152 -> [w411]
    tunnel: w151 -> [w410]
    tunnel: w150 -> [w405]
    tunnel: [w408] -> w149
    tunnel: [w407] -> w148
    tunnel: w143 -> [w406]
    tunnel: [w405] -> w142
    tunnel: w137 -> [w404]
    tunnel: [w404] -> w136
    tunnel: w14 -> [w403]
    tunnel: [w403] -> w77
    tunnel: w12 -> [w402]
    tunnel: [w402] -> w75
    tunnel: w49 -> [w401]
    tunnel: [w401] -> w51
    tunnel: w46 -> [w400]
    tunnel: [w400] -> w45
    tunnel: [w487] -> w361
    tunnel: w356 -> [w486]
    tunnel: [w486] -> w355
    tunnel: w354 -> [w485]
    tunnel: [w485] -> w353
    tunnel: w352 -> [w484]
    tunnel: [w484] -> w351
    tunnel: w350 -> [w483]
    tunnel: [w483] -> w349
    tunnel: [w477] -> w348
    tunnel: [w476] -> w347
    tunnel: [w482] -> w346
    tunnel: [w481] -> w345
    tunnel: w344 -> [w481]
    tunnel: [w480] -> w331
    tunnel: w334 -> [w480]
    tunnel: [w479] -> w332
    tunnel: w333 -> [w479]
    tunnel: [w478] -> w329
    tunnel: w328 -> [w478]
    tunnel: w326 -> [w475]
    tunnel: w324 -> [w474]
    tunnel: w274 -> [w473]
    tunnel: [w473] -> w273
    tunnel: w269 -> [w450]
    tunnel: w253 -> [w471]
    tunnel: w251 -> [w470]
    tunnel: [w469] -> w250
    tunnel: [w468] -> w249
    tunnel: [w467] -> w248
    tunnel: w247 -> [w467]
    tunnel: w246 -> [w466]
    tunnel: [w466] -> w245
    tunnel: w244 -> [w465]
    tunnel: [w465] -> w243
    tunnel: w242 -> [w464]
    tunnel: [w464] -> w241
    tunnel: [w463] -> w214
    tunnel: [w462] -> w213
    tunnel: w212 -> [w461]
    tunnel: [w461] -> w211
    tunnel: w210 -> [w460]
    tunnel: [w460] -> w209
    tunnel: w207 -> [w459]
    tunnel: w205 -> [w458]
    tunnel: w201 -> [w457]
    tunnel: [w457] -> w200
    tunnel: w198 -> [w456]
    tunnel: [w456] -> w197
    tunnel: w149 -> [w455]
    tunnel: w148 -> [w454]
    tunnel: [w453] -> w147
    tunnel: [w452] -> w146
    tunnel: [w451] -> w141
    tunnel: w142 -> [w451]
    tunnel: [w449] -> w139
    tunnel: [w448] -> w138
    tunnel: w136 -> [w446]
    tunnel: w77 -> [w445]
    tunnel: [w445] -> w76
    tunnel: w75 -> [w444]
    tunnel: [w444] -> w2
    tunnel: w51 -> [w443]
    tunnel: [w443] -> w50
    tunnel: w45 -> [w442]
    tunnel: [w442] -> w44
    frame #0 {
      # "# of stimulators"
      n131 = call <vilib>:"DAQmx Start Task.vi"("task/channels in"=w434, "error in"=w433) -> ("task out"=w432:refnum<k21>, "error out"=w431:errorcluster)  [unwired: 12 in]
      n132 = call <vilib>:"IMAQdx Configure Grab.vi"("error in"=w441, "Session In"=w440) -> ("error out"=w437:errorcluster, "Session Out"=w438:T5)  [unwired: 8 in]
      n133 = call <vilib>:"IMAQdx Start Acquisition.vi"("error in"=w414, "Session In"=w415) -> ("error out"=w418:errorcluster, "Session Out"=w419:T5)  [unwired: 8 in]
      n134 = call-dynamic "record.vi"("Camera in"=w411, "num_images"=w406, "record_mode"=T13."pcoraw", "file_path"=w405, "error in (no error)"=w410) -> ("Camera out"=w408:refnum<class "Camera.lvclass">, "error out"=w407:errorcluster)  [unwired: 9 in]
    }
    frame #1 {
      n135 = call <vilib>:"DAQmx Start Task.vi"("task/channels in"=w459, "error in"=w458) -> ("task out"=w463:refnum<k21>, "error out"=w462:errorcluster)  [unwired: 12 in]
      n136 = local write "CBV Camera"(FALSE ("Finished Acquiring")) -> ()
      n137 = Tick Count (ms)() -> (millisecond timer value=w487:u32)
      n138 = call-dynamic "waitForFirstImage.vi"("error in (no error)"=w454, "Camera in"=w455) -> ("error out"=w452:errorcluster, "Camera out"=w453:refnum<class "Camera.lvclass">)  [unwired: 8 in]
      n139 = call <vilib>:"DAQmx Start Task.vi"("task/channels in"=w471, "error in"=w470) -> ("task out"=w469:refnum<k21>, "error out"=w468:errorcluster)  [unwired: 12 in]
      n140 = Tick Count (ms)() -> (millisecond timer value=w482:u32)
      n141 = call-poly <vilib>:"DAQmx Write.vi"("task/channels in"=w446, "data"=TRUE, "error in"=w450) -> ("task out"=w449:refnum<k21>, "error out"=w448:errorcluster)  [unwired: 10 in, 1 out]
      n142 = call <vilib>:"DAQmx Start Task.vi"("task/channels in"=w475, "error in"=w474) -> ("task out"=w477:refnum<k21>, "error out"=w476:errorcluster)  [unwired: 12 in]
    }
  }
  n143 = Greater?(x=w5, y=w2) -> (0:w6:bool)
  n144 = Absolute Value(x=w2) -> (abs(x)=w1:dbl)
  n145 = case shown="True" w6 {
    tunnel: w1 -> [w489 w490]
    tunnel: w5 -> [w488 w491]
    tunnel: [w489 w491] -> w4
    tunnel: [w488 w490] -> w3
    frame False {
      # "If stim offset is positive or zero, stim and squeeze are routed as originally wired"
    }
    frame True {
      # "If stim offset is strictly negative, stim precedes squeeze"
    }
  }
  n146 = To Long Integer(number=w273) -> (32bit integer=w272:i32)
  n147 = while {
    tunnel: [w549] -> w127
    tunnel: w348 -> [w549]
    tunnel: [w548] -> w126
    tunnel: w347 -> [w548]
    tunnel: w346 -> [w547]
    tunnel: w345 -> [w500]
    tunnel: w139 -> [w544]
    tunnel: [w544] -> w131
    tunnel: [w543] -> w130
    tunnel: w138 -> [w543]
    tunnel: [w542] -> w129
    tunnel: [w541] -> w128
    tunnel: w250 -> [w540]
    tunnel: w249 -> [w539]
    tunnel: w20 -> [w538]
    tunnel: w248 -> [w514]
    tunnel: w245 -> [w537]
    tunnel: w243 -> [w511]
    tunnel: w241 -> [w512]
    tunnel: w147 -> [w536]
    tunnel: w146 -> [w535]
    tunnel: [w524] -> w133
    tunnel: [w525] -> w134
    tunnel: w143 -> [w523]
    tunnel: w141 -> [w519]
    tunnel: [w519] -> w132
    tunnel: w20 -> [w516]
    tunnel: w76 -> [w515]
    tunnel: w20 -> [w513]
    tunnel: w4 -> [w507]
    tunnel: w50 -> [w502]
    tunnel: w44 -> [w501]
    tunnel: w3 -> [w492]
    stop <- w546 stop-if-true
    # "Record from PCO"
    # "Write T/F \nto Solenoid\nArray"
    # "Track Time elapsed during trial"
    # "Record PCO"
    n148 = Tick Count (ms)() -> (millisecond timer value=w550:u32)
    n149 = call-dynamic "isRecording.vi"("Camera in"=w536, "error in (no error)"=w535) -> ("Camera out"=w534:refnum<class "Camera.lvclass">, "recording"=→"PCO Recording":bool, "error out"=w533:errorcluster)  [unwired: 11 in]
    n150 = Subtract(x=w550, y=w547) -> (x-y=w498:u32)
    n151 = call-dynamic "getRecordedImageCount.vi"("Camera in"=w534, "error in (no error)"=w533) -> ("Camera out"=w527:refnum<class "Camera.lvclass">, "recorded_image_count"=w505:u32, "error out"=w526:errorcluster)  [unwired: 11 in]
    "Recorded Images" <- w505
    n152 = Greater?(x=w505, y=w516) -> (0:w506:bool)
    n153 = case shown="True" w506 {
      tunnel: w514 -> [_ w578]
      tunnel: w515 -> [_ w554]
      tunnel: w513 -> [_ w573]
      tunnel: w512 -> [_ w575]
      tunnel: w505 -> [_ w574]
      tunnel: [FALSE ("Boolean") w560] -> w510
      tunnel: w511 -> [_ w571]
      tunnel: w502 -> [_ w558]
      tunnel: w501 -> [_ w557]
      tunnel: w492 -> [_ w553]
      frame False {
      }
      frame True {
        # "if control,\nmodulate stimulus"
        # "Track Solenoid\nOrder"
        # "Squeezes"
        n154 = Subtract(x=w574, y=w573) -> (x-y=w572:dbl)
        n155 = Quotient & Remainder(x=w572, y=w578) -> (x-y*floor(x/y)=w559:dbl, floor(x/y)=w576:dbl)
        n156 = Quotient & Remainder(x=w576, y=w575) -> (x-y*floor(x/y)=w577:dbl)  [unwired: 1 out]
        n157 = Add(x=w553, y=0.0 ("lower limit")) -> (x+y=w555:dbl)
        n158 = Add(x=w554, y=w553) -> (x+y=w552:dbl)
        n159 = Index Array(array=w571, index=w577) -> (element=w563:dbl)
        n160 = Not Equal?(x=w563, y=0.0) -> (x != y?=w566:bool)
        n161 = In Range and Coerce(upper limit=w552, x=w559, lower limit=w555) -> (In Range?=w570:bool)  [unwired: 1 out]
        n162 = Equal?(x=4.0 ("lower limit"), y=w563) -> (x = y?=w562:bool)
        n163 = Not Equal?(x=w563, y=3.0) -> (x != y?=w567:bool)
        n164 = And(x=w566, y=w567) -> (x .and. y?=w565:bool)
        n165 = And(x=w570, y=w565) -> (x .and. y?=w561:bool)
        n166 = case shown="True" w562 {
          tunnel: w561 -> [w579 w581]
          tunnel: [w579 w580] -> w560
          tunnel: w559 -> [_ w586]
          tunnel: w558 -> [_ w585]
          tunnel: w557 -> [_ w583]
          frame False {
          }
          frame True {
            n167 = Quotient & Remainder(x=w586, y=w585) -> (x-y*floor(x/y)=w584:dbl)  [unwired: 1 out]
            n168 = Less Or Equal?(x=w584, y=w583) -> (x <= y?=w582:bool)
            n169 = And(x=w582, y=w581) -> (x .and. y?=w580:bool)
          }
        }
      }
    }
    n170 = case shown="True" w506 {
      tunnel: w514 -> [_ w611]
      tunnel: w537 -> [_ w599]
      tunnel: w538 -> [_ w606]
      tunnel: w512 -> [_ w608]
      tunnel: w511 -> [_ w607]
      tunnel: w505 -> [_ w602]
      tunnel: [FALSE w603] -> w509
      tunnel: w507 -> [_ w600]
      frame False {
      }
      frame True {
        # "Track ISI"
        # "Track Solenoid\nOrder"
        # "Puffs"
        n171 = Subtract(x=w602, y=w606) -> (x-y=w605:dbl)
        n172 = Quotient & Remainder(x=w605, y=w611) -> (x-y*floor(x/y)=w612:dbl, floor(x/y)=w609:dbl)
        n173 = Quotient & Remainder(x=w609, y=w608) -> (x-y*floor(x/y)=w610:dbl)  [unwired: 1 out]
        n174 = Index Array(array=w607, index=w610) -> (element=w591:dbl)
        n175 = Add(x=w600, y=0.0 ("lower limit")) -> (x+y=w597:dbl)
        n176 = Add(x=w600, y=w599) -> (x+y=w598:dbl)
        n177 = Not Equal?(x=w591, y=1.0) -> (x != y?=w594:bool)
        n178 = In Range and Coerce(upper limit=w598, x=w612, lower limit=w597) -> (In Range?=w604:bool)  [unwired: 1 out]
        n179 = Not Equal?(x=w591, y=3.0) -> (x != y?=w593:bool)
        n180 = And(x=w594, y=w593) -> (x .and. y?=w589:bool)
        n181 = Not Equal?(x=w591, y=4.0) -> (x != y?=w590:bool)
        n182 = And(x=w589, y=w590) -> (x .and. y?=w588:bool)
        n183 = And(x=w604, y=w588) -> (x .and. y?=w603:bool)
      }
    }
    n184 = Greater Or Equal?(x=w505, y=w523) -> (x >= y?=w522:bool)
    n185 = Divide(x=w498, y=1000.0) -> (x/y=w494:dbl)
    "Time Elapsed (s)" <- w494
    n186 = local read "Image"() -> (w504:T3)
    n187 = Divide(x=w505, y=w494) -> (x/y=→"PCO Frame Rate":dbl)
    n188 = call-dynamic "image.vi"("Camera in"=w527, "data_format"=T14."Mono16", "image_index"=u32 4294967295 ("dwImgIdx"), "error in (no error)"=w526) -> ("Camera out"=w524:refnum<class "Camera.lvclass">, "raw_image (U16)"=w528:u16[][], "error out"=w525:errorcluster)  [unwired: 4 in, 5 out]
    n189 = Divide(x=w500, y=60.0) -> (x/y=w496:dbl)
    n190 = local write "Stop"("Stop") -> ()
    n191 = Divide(x=w494, y=60.0) -> (x/y=w493:dbl)
    n192 = call "IMAQ ArrayToImage"("Image Pixels (U16)"=w528, "Image"=w504) -> ("error out"=w530:errorcluster, "Image Out"=w503:T3)  [unwired: 8 in]
    n193 = Bundle(w496, w493) -> (→"Trial Time Elapsed (Min)":cluster{dbl, dbl})  [unwired: 1 in]
    n194 = local write "Image"(w503) -> ()
    n195 = Unbundle By Name(w530) -> ("status"=w521:bool)
    n196 = Build Array(w509, w510, w509) -> (w508:bool[])
    "Solenoids" <- w508
    n197 = Unbundle By Name(w525) -> ("status"=w520:bool)
    n198 = Compound Arithmetic op=OR("Stop", w522, w521, w520) -> (w546:bool)
    "CBV Camera" <- w546
    n199 = call-poly <vilib>:"DAQmx Write.vi"("task/channels in"=w540, "data"=w508, "error in"=w539) -> ("task out"=w542:refnum<k21>, "error out"=w541:errorcluster)  [unwired: 10 in, 1 out]
  }
  n200 = while {
    tunnel: w361 -> [w625]
    tunnel: w355 -> [w618]
    tunnel: w353 -> [w624]
    tunnel: w351 -> [w623]
    tunnel: w349 -> [w619]
    tunnel: [w622] -> w123
    tunnel: [w621] -> w125
    tunnel: [w620] -> w124
    i -> [w617]
    stop <- w626 stop-if-true
    # "Record Webcam"
    n201 = Quotient & Remainder(x=w617, y=2) -> (x-y*floor(x/y)=w615:i32)  [unwired: 1 out]
    n202 = Less Or Equal?(x=w615, y=0) -> (x <= y?=w613:bool)
    n203 = case shown="True" w613 {
      tunnel: w625 -> [_ w640]
      tunnel: w624 -> [w629 w639]
      tunnel: w623 -> [w628 w635]
      tunnel: [w629 w634] -> w622
      tunnel: [w628 w632] -> w621
      tunnel: [w627 w630] -> w620
      tunnel: w619 -> [w627 w630]
      tunnel: w618 -> [_ w638]
      tunnel: w617 -> [_ w637]
      frame False {
      }
      frame True {
        n204 = Tick Count (ms)() -> (millisecond timer value=w643:u32)
        n205 = Subtract(x=w643, y=w640) -> (x-y=w644:u32)
        n206 = Divide(x=w644, y=u32 1000) -> (x/y=w636:dbl)
        n207 = call "WebCam Grab_FLIR_trig.vi"("Session In"=w639, "Image In"=w638, "Buffer Number In"=w637, "Trial Time"=w636, "AVI Refnum"=w630, "error in"=w635) -> ("Session Out"=w634:T5, "WebCam Img Out"=→"WebCam":T3, "Buffer Number Out"=w631:u32, "error out"=w632:errorcluster)  [unwired: 10 in]
        n208 = call <vilib>:"Calculate Frames per Second.vi"("Update Interval (ms)"=u32 5000, "Buffer Number"=w631) -> ("Processed Frames/s"=→"Actual WebCam Frame Rate":dbl)  [unwired: 7 in, 2 out]
      }
    }
    n209 = local read "CBV Camera"() -> (w626:bool)
  }
  n210 = while {
    tunnel: w214 -> [w665]
    tunnel: [w666] -> w119
    tunnel: w213 -> [w666]
    tunnel: [w665] -> w120
    tunnel: [w648] -> w121
    tunnel: [w650] -> w114
    tunnel: [w664] -> w113
    tunnel: w211 -> [w663]
    tunnel: w209 -> [w662]
    tunnel: w200 -> [w661]
    tunnel: w197 -> [w660]
    shift-right: [w659] -> w11
    shift-left: u32 0 ("Buffer Number Out") -> [w658]
    shift-right: [w657] -> w8
    shift-left: u32 0 ("New Lost") -> [w656]
    shift-right: [w655] -> w10
    shift-left: u32[] [] ("NewBuffNum") -> [w654]
    shift-right: [w653] -> w9
    shift-left: u32[] [] ("NewNumLost") -> [w652]
    stop <- w651 stop-if-true
    # "Track Dropped Frames"
    # "Record auxiliary camera (whiskers/pupil depending on setup)"
    n211 = call <vilib>:"IMAQdx Get Image.vi"("Buffer Number Mode (Next)"=IMAQdx_Buffer_Number_Mode."Next", "error in"=w662, "Image In"=w661, "Session In"=w663) -> ("error out"=w673:errorcluster, "Buffer Number Out"=w659:u32, "Image Out"=w646:T3, "Session Out"=w648:T5)  [unwired: 4 in]
    "Last Whisk\nBuffer" <- w659
    "Pupil" <- w646
    n212 = call "Track Dropped Frames_atw1.vi"("NumLost"=w652, "BuffNum"=w654, "Curr Buffer"=w659, "Prev Lost"=w656, "Prev Buffer"=w658) -> ("New Lost"=w657:u32, "NewNumLost"=w653:u32[], "NewBuffNum"=w655:u32[])  [unwired: 4 in]
    n213 = local read "CBV Camera"() -> (w647:bool)
    n214 = call "IMAQ ImageToArray"("error in (no error)"=w673, "Image"=w646) -> ("error out"=w672:errorcluster, "Image Pixels (U8)"=w671:u8[][])  [unwired: 2 in, 3 out]
    n215 = call <vilib>:"Calculate Frames per Second.vi"("Update Interval (ms)"=u32 2000, "Buffer Number"=w659) -> ("Processed Frames/s"=→"Actual WhiskCam\nFrame Rate":dbl)  [unwired: 7 in, 2 out]
    n216 = Write to Binary File(file (use dialog)=w660, data=w671, error in=w672, 5:FALSE ("prepend array or string size? (T)"), 9:T15."little-endian" ("byte order (0:big-endian, network order)")) -> (refnum out=w664:refnum<file>, error out=w650:errorcluster)  [unwired: 1 in, 1 out]
    n217 = Unbundle By Name(w650) -> ("status"=w649:bool)
    n218 = Or(x=w649, y=w647) -> (x .or. y?=w651:bool)
  }
  "Buffer Number Out" <- w11
  "NewBuffNum" <- w10
  "NewNumLost" <- w9
  "New Lost" <- w8
  n219 = while {
    tunnel: w332 -> [w694]
    tunnel: w331 -> [w693]
    tunnel: w329 -> [w692]
    tunnel: [w691] -> w115
    tunnel: [w675] -> w116
    tunnel: [w690] -> w122
    shift-right: [w682] -> _
    shift-left: 0 -> [w683]
    tunnel: w272 -> [w681]
    stop <- w677 stop-if-true
    # "Record Analog Data"
    n220 = call-poly <vilib>:"DAQmx Read.vi"("task/channels in"=w693, "error in"=w694) -> ("task out"=w690:refnum<k21>, "data"=w688:waveform(dbl)[], "error out"=w680:errorcluster)  [unwired: 11 in]
    n221 = Index Array(array=w688, index=0) -> (element=w686:waveform(dbl))
    n222 = Unbundle By Name(w686) -> ("Y"=w685:dbl[])
    n223 = Array Size(array=w685) -> (size(s)=w684:i32)
    n224 = local read "Stop"() -> (w678:bool)
    n225 = local read "CBV Camera"() -> (w676:bool)
    n226 = Add(x=w684, y=w683) -> (x+y=w682:i32)
    "Analog acquisition length" <- w682
    n227 = Greater Or Equal?(x=w682, y=w681) -> (x >= y?=w679:bool)
    n228 = TDMS Write(0:w692, 5:"Analog Data" ("group name in (Untitled)"), 9:w688, 11:w680) -> (4:w691:refnum<k34>, 15:w675:errorcluster)  [unwired: 2 in, 2 out]
    n229 = Compound Arithmetic op=OR(w675, w679, w678, w676) -> (w677:bool)
    "Analog Data" <- w677
  }
  n230 = while {
    shift-right: [w722] -> _
    shift-left: enum16{"Close all devices", "Move files"}."Close all devices" ("Enum") -> [w723]
    tunnel: w133 -> [w720]
    tunnel: w132 -> [w719]
    tunnel: w131 -> [w718]
    tunnel: w130 -> [w717]
    tunnel: w129 -> [w716]
    tunnel: w128 -> [w715]
    tunnel: w127 -> [w714]
    tunnel: w126 -> [w713]
    tunnel: w124 -> [w711]
    tunnel: w123 -> [w710]
    tunnel: w122 -> [w709]
    tunnel: w121 -> [w706]
    tunnel: w120 -> [w705]
    tunnel: w119 -> [w704]
    tunnel: w118 -> [w703]
    shift-right: [w696] -> w110
    shift-left: w125 -> [w712]
    tunnel: "Target Path" -> [w702]
    tunnel: w115 -> [w701]
    shift-right: [w697] -> w111
    shift-left: w116 -> [w708]
    tunnel: w113 -> [w700]
    shift-right: [w698] -> w112
    shift-left: w114 -> [w707]
    shift-right: [w695] -> w109
    shift-left: w134 -> [w721]
    stop <- w699 stop-if-true
    # "Close, save & exit"
    n231 = case shown="\"Close all devices\", Default" w723 {
      tunnel: [enum16{"Close all devices", "Move files"}."Move files" ("Enum") enum16{"Close all devices", "Move files"}."Close all devices" ("Enum")] -> w722
      tunnel: w721 -> [w757 w760]
      tunnel: w720 -> [w756 _]
      tunnel: w719 -> [_ w782]
      tunnel: w718 -> [w751 _]
      tunnel: w717 -> [w749 _]
      tunnel: w716 -> [w727 _]
      tunnel: w715 -> [w725 _]
      tunnel: w714 -> [w746 _]
      tunnel: w713 -> [w745 _]
      tunnel: w712 -> [w743 w780]
      tunnel: w711 -> [w744 _]
      tunnel: w710 -> [w742 _]
      tunnel: w709 -> [w741 _]
      tunnel: w708 -> [w740 w772]
      tunnel: w707 -> [w738 w767]
      tunnel: w706 -> [w737 _]
      tunnel: w705 -> [w736 _]
      tunnel: w704 -> [w735 _]
      tunnel: w703 -> [_ w781]
      tunnel: w702 -> [_ w768]
      tunnel: w701 -> [_ w759]
      tunnel: w700 -> [_ w769]
      tunnel: [FALSE TRUE] -> w699
      tunnel: [w730 w764] -> w698
      tunnel: [w731 w763] -> w697
      tunnel: [w732 w762] -> w696
      tunnel: [w729 w761] -> w695
      frame "Close all devices", Default {
        # "occasionally the trial\nends with the puffer left on\nunless we explicitly write falses\nto all stim lines"
        # "next loop: handle files"
        # "Stop PCO recording and release resources\n\nNOTE: IF THIS IS NOT RUN AT \nTHE END OF EVERY TRIAL, THE\nCAMERA WILL BE DEADLOCKED\nIN A RECORDING SESSION AND \nYOU WILL HAVE TO RESTART THE CAMERA\nAND/OR COMPUTER TO RESET IT\n\n(this wastes a lot of time)"
        # "Stop & clear start trigger"
        # "Stop & clear sensory stim output"
        # "Stop counter task"
        # "Close video object\n& release resources"
        # "Close webcam AVI"
        # "Close video object & release resources"
        # "Stop camera acquisition"
        # "Stop & clear analog acquisition task"
        # "-1 will release the buffer."
        n232 = call-dynamic "close.vi"("error in (no error)"=w757, "Camera in"=w756) -> ("error out"=w729:errorcluster)  [unwired: 9 in]
        n233 = call <vilib>:"DAQmx Stop Task.vi"("task/channels in"=w746, "error in"=w745) -> ()  [unwired: 12 in, 2 out]
        n234 = call <vilib>:"IMAQdx Close Camera.vi"("error in"=w738, "Session In"=w737) -> ("error out"=w730:errorcluster)  [unwired: 9 in]
        n235 = call-poly <vilib>:"DAQmx Write.vi"("task/channels in"=w751, "data"=FALSE, "error in"=w749) -> ("task out"=w752:refnum<k21>, "error out"=w754:errorcluster)  [unwired: 10 in, 1 out]
        n236 = call <vilib>:"DAQmx Stop Task.vi"("task/channels in"=w736, "error in"=w735) -> ()  [unwired: 12 in, 2 out]
        n237 = call <vilib>:"DAQmx Stop Task.vi"("task/channels in"=w741, "error in"=w740) -> ("task out"=w739:refnum<k21>, "error out"=w734:errorcluster)  [unwired: 12 in]
        n238 = call "IMAQ AVI2 Close"("error in (no error)"=w743, "AVI Refnum"=w744) -> ("error out"=w732:errorcluster)  [unwired: 9 in]
        n239 = call <vilib>:"IMAQdx Close Camera.vi"("error in"=w743, "Session In"=w742) -> ()  [unwired: 9 in, 1 out]
        n240 = call-poly <vilib>:"DAQmx Write.vi"("task/channels in"=w727, "data"=bool[] [FALSE, FALSE, FALSE], "error in"=w725) -> ("task out"=w726:refnum<k21>, "error out"=w724:errorcluster)  [unwired: 10 in, 1 out]
        n241 = call <vilib>:"DAQmx Stop Task.vi"("task/channels in"=w752, "error in"=w754) -> ("task out"=w753:refnum<k21>, "error out"=w755:errorcluster)  [unwired: 12 in]
        n242 = call <vilib>:"DAQmx Clear Task.vi"("task in"=w739, "error in"=w734) -> ("error out"=w731:errorcluster)  [unwired: 13 in]
        n243 = call <vilib>:"DAQmx Clear Task.vi"("task in"=w753, "error in"=w755) -> ()  [unwired: 13 in, 1 out]
        n244 = call <vilib>:"DAQmx Stop Task.vi"("task/channels in"=w726, "error in"=w724) -> ("task out"=w748:refnum<k21>, "error out"=w747:errorcluster)  [unwired: 12 in]
        n245 = call <vilib>:"DAQmx Clear Task.vi"("task in"=w748, "error in"=w747) -> ()  [unwired: 13 in, 1 out]
      }
      frame "Move files" {
        # "(shouldn't run)"
        n246 = Path To String(path=w782) -> (string=w784:string)
        n247 = Close File(refnum=w769, error in=w767) -> (path=w770:path, error out=w771:errorcluster)
        n248 = Concatenate Strings(w784, "_Cam01.pcoraw" ("string")) -> (w785:string)
        n249 = TDMS Close(8:w772, 11:w759) -> (0:w774:errorcluster, 3:w776:path)
        n250 = String To Path(string=w785) -> (path=w786:path)
        n251 = Move(source path=w781, error in=w780, 10:w768) -> (error out=w762:errorcluster)  [unwired: 2 in, 2 out]
        n252 = TDMS Defragment(4:w774, 7:w776) -> (0:w779:errorcluster)
        n253 = Move(source path=w770, error in=w771, 10:w768) -> (error out=w764:errorcluster)  [unwired: 2 in, 2 out]
        n254 = Path To String(path=w776) -> (string=w775:string)
        n255 = Move(source path=w786, error in=w760, 10:w768) -> (error out=w761:errorcluster)  [unwired: 2 in, 2 out]
        n256 = Concatenate Strings(w775, "_index" ("string")) -> (w777:string)
        n257 = String To Path(string=w777) -> (path=w778:path)
        n258 = Move(source path=w776, error in=w779, 10:w768) -> (error out=w763:errorcluster)  [unwired: 2 in, 2 out]
        n259 = Move(source path=w778, error in=w779, 10:w768) -> ()  [unwired: 2 in, 3 out]
      }
    }
  }
  n260 = call <vilib>:"Simple Error Handler.vi"("error in (no error)"=w112) -> ()  [unwired: 1 in, 8 out]
  n261 = call <vilib>:"Simple Error Handler.vi"("error in (no error)"=w109) -> ()  [unwired: 1 in, 8 out]
  n262 = call <vilib>:"Simple Error Handler.vi"("error in (no error)"=w110) -> ()  [unwired: 1 in, 8 out]
  n263 = call <vilib>:"Simple Error Handler.vi"("error in (no error)"=w111) -> ()  [unwired: 1 in, 8 out]
